vi "LVDimInterface.application example serv command_integer_double.vi"() -> ()   [LabVIEW 2012, in "LVDimInterface.lvlib"]
doc: "This VI implements a DIM server, that receives commands via a message queue."
uses:
  LVDimInterface.lvlib
  LVDimInterface.dis_add_command_queue.vi
panel:
  out "error out":errorcluster
  out "double":dbl
  out "integer":i32
  out "callBackID":i32=-1
  in  "serverName":string="test27"
  out "received commands":i32=-1
  out "loop counter":i32
  in  "stop":bool
  in  "commandName":string="testCommand2"
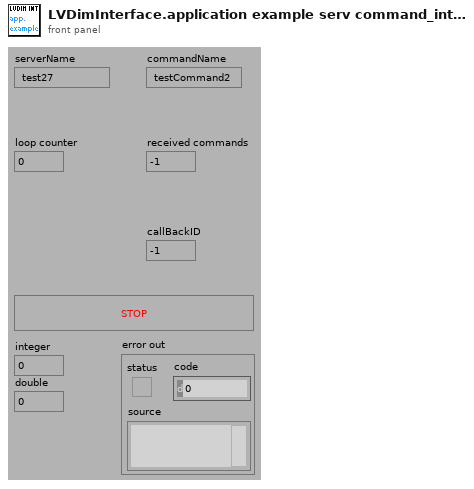
[diagram p1: front panel]
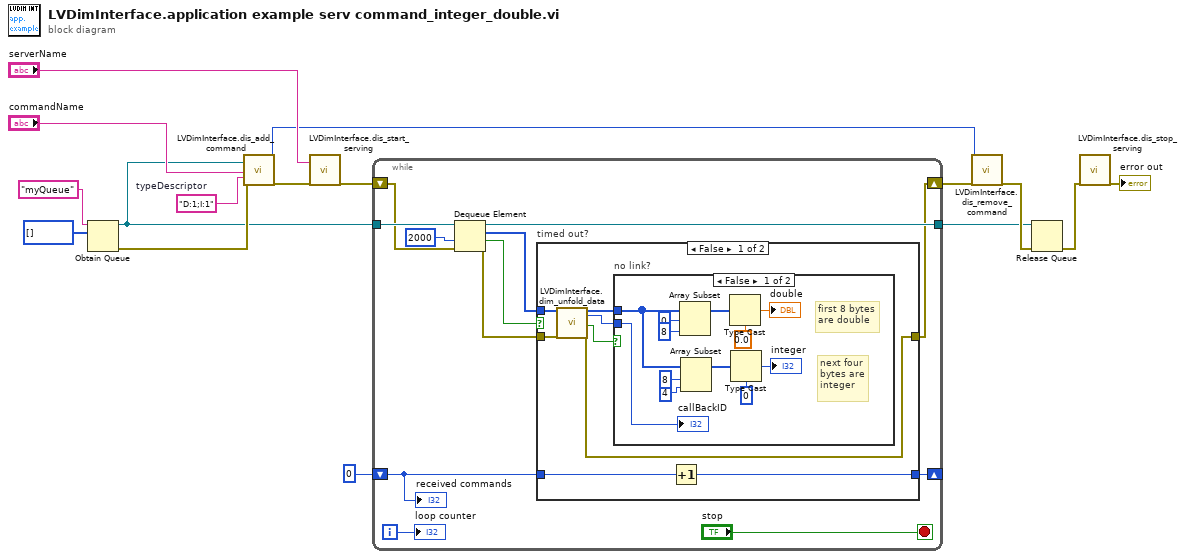
[diagram p0: block diagram]
diagram:
  w6 = "D:1;I:1"  # typeDescriptor
  n1 = Obtain Queue(name (unnamed)="myQueue" ("test1"), element data type=i8[] []) -> (queue out=w1:refnum<queue>, error out=w4:errorcluster)  [unwired: 3 in, 1 out]
  n2 = call-poly "LVDimInterface.dis_add_command.vi"("queueRef"=w1, "commandName"="commandName", "typeDescriptor"=w6, "error in (no error)"=w4) -> ("commandID"=w10:i32, "error out"=w12:errorcluster)  [unwired: 14 in]
  n3 = call "LVDimInterface.dis_start_serving.vi"("serverName"="serverName", "error in (no error)"=w12) -> ("error out"=w14:errorcluster)  [unwired: 16 in, 1 out]
  n4 = while {
    tunnel: w1 -> [w27]
    shift-right: [w21] -> _
    shift-left: 0 -> [w22]
    tunnel: [w20] -> w5
    shift-right: [w17] -> w8
    shift-left: w14 -> [w18]
    i -> [w25]
    stop <- "stop" stop-if-true
    n5 = Dequeue Element(queue=w27, timeout in ms (-1)=2000, error in (no error)=w18) -> (queue out=w20:refnum<queue>, element=w24:i8[], timed out?=w23:bool, error out=w19:errorcluster)
    n6 = case "timed out?" shown="False" w23 {
      tunnel: w24 -> [w34 _]
      tunnel: [w35 w50] -> w21
      tunnel: w22 -> [w36 w50]
      tunnel: w19 -> [w31 w49]
      tunnel: [w30 w49] -> w17
      frame False {
        n7 = call "LVDimInterface.dim_unfold_data.vi"("rawData"=w34, "error in (no error)"=w31) -> ("data"=w29:i8[], "callBackID"=w33:i32, "no link"=w32:bool, "error out"=w30:errorcluster)  [unwired: 14 in]
        n8 = case "no link?" shown="False" w32 {
          tunnel: w33 -> [w48 _]
          tunnel: w29 -> [w37 _]
          frame False {
            # "next four\nbytes are\ninteger"
            # "first 8 bytes\nare double"
            n9 = Array Subset(array=w37, index=0, length=8) -> (w42:i8[])
            n10 = Array Subset(array=w37, index=8, length=4) -> (w45:i8[])
            n11 = Type Cast(type=0.0, x=w42) -> (*(type *) &x=→"double":dbl)
            n12 = Type Cast(type=0, x=w45) -> (*(type *) &x=→"integer":i32)
            "callBackID" <- w48
          }
          frame True {
          }
        }
        n13 = Increment(x=w36) -> (x+1=w35:i32)
      }
      frame True {
      }
    }
    "loop counter" <- w25
    "received commands" <- w22
  }
  n14 = call "LVDimInterface.dis_remove_command.vi"("commandID"=w10, "error in (no error)"=w8) -> ("error out"=w9:errorcluster)  [unwired: 17 in]
  n15 = Release Queue(queue=w5, error in (no error)=w9) -> (error out=w3:errorcluster)  [unwired: 1 in, 2 out]
  n16 = call "LVDimInterface.dis_stop_serving.vi"("error in (no error)"=w3) -> ("error out"=→"error out":errorcluster)  [unwired: 18 in]
